vi "BallToGoalSkillVss.vi"(8 "error in (no error)":errorcluster, 9 "Game":refnum<class "Game.lvclass">, 10 "Robot in":refnum<class "Robot.lvclass">, 11 "BallToGoalSkillVSS in":refnum<class "BallToGoalSkillVSS.lvclass">) -> (0 "error out":errorcluster, 2 "Robot out":refnum<class "Robot.lvclass">, 3 "BallToGoalSkillVSS out":refnum<class "BallToGoalSkillVSS.lvclass">)   [LabVIEW 2020, in "BallToGoalSkillVSS.lvclass"]
uses:
  BallToGoalSkillVSS.lvclass
  Robot_class/Robot.lvclass
  C:/Users/pedro/Desktop/SSL_AI/Object_class/Object.lvclass
  Game_class/Game.lvclass
  Game_class/Game.lvclass/Game.ctl
  Object_class/Object.lvclass/Object.ctl
  Robot_class/Robot.lvclass/Robot.ctl
  Game_class/Read BallRef.vi
  Game_class/Read FieldRef.vi
  Object_class/Read x.vi
  Object_class/Read y.vi
  Object_class/Write x.vi
  Object_class/Write y.vi
  Robot_class/Write dest_orientation.vi
  Ball_class/Ball.lvclass
  Field_class/Field.lvclass
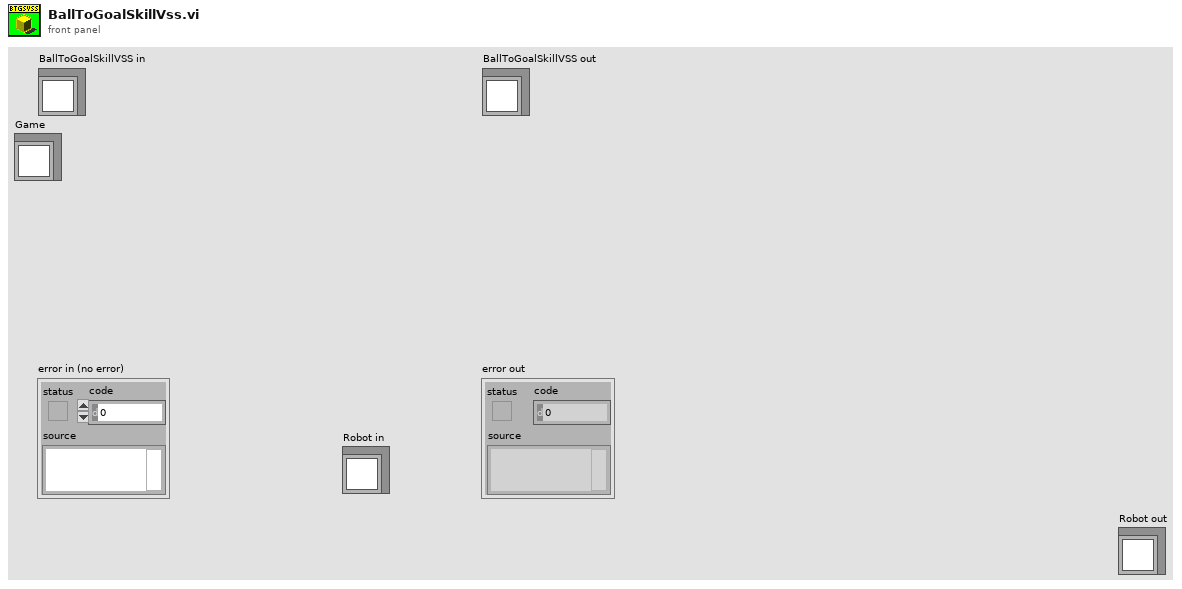
[diagram p1: front panel]
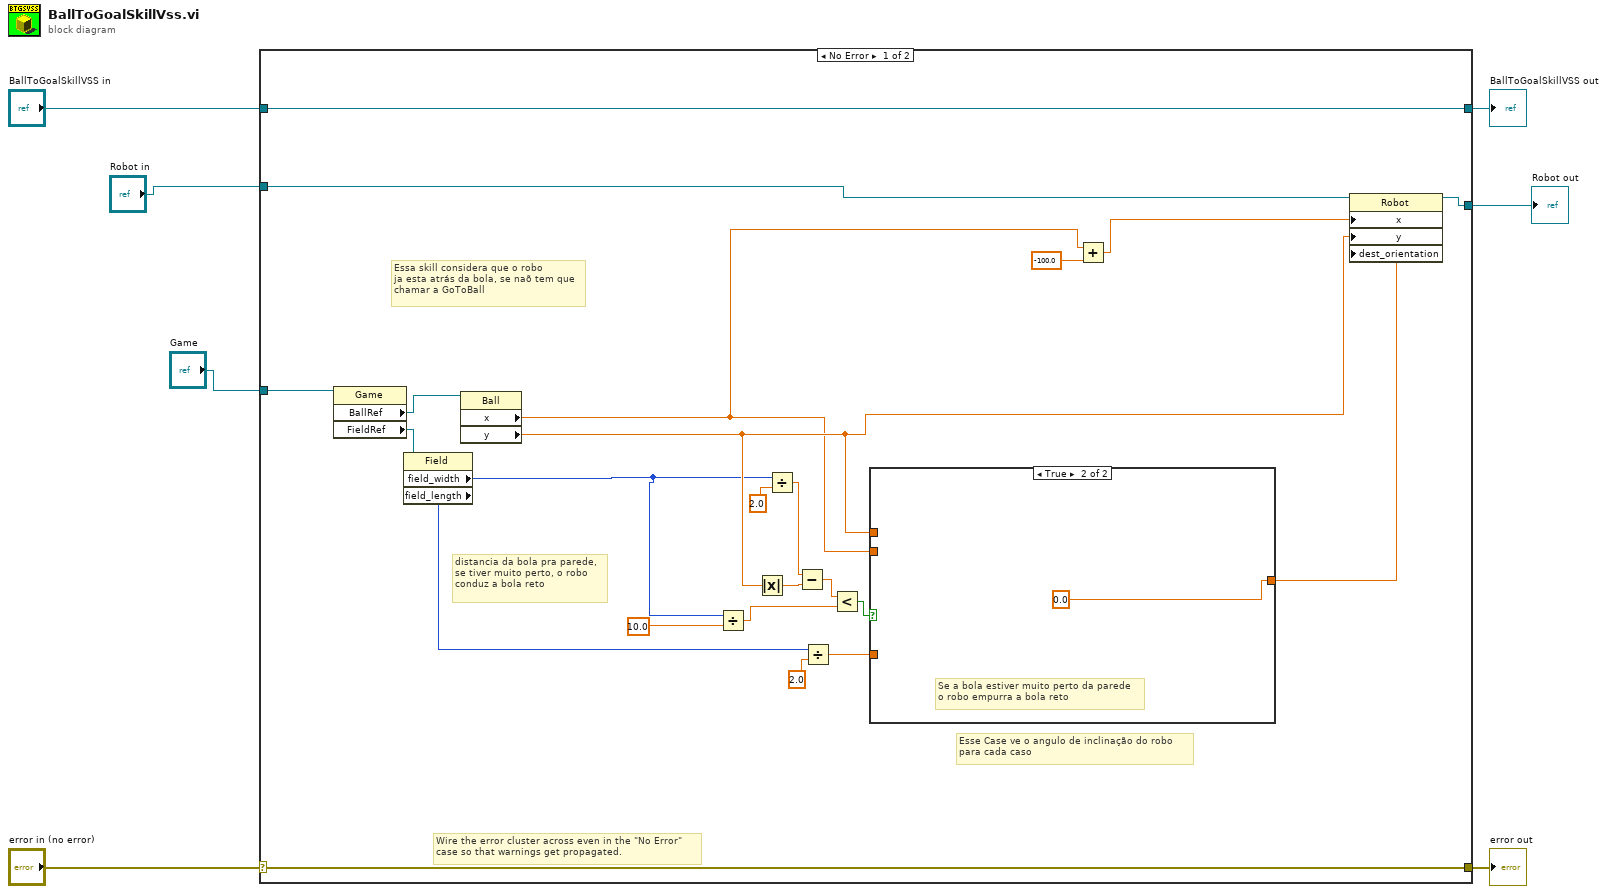
[diagram p0: block diagram]
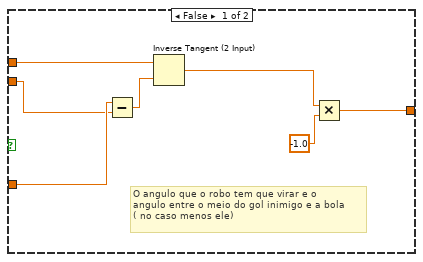
[diagram p2: hidden frame]
diagram:
  n1 = case shown="No Error" "error in (no error)" {
    selector: "error in (no error)" -> [w29 w41]
    tunnel: [w29 w41] -> w6
    tunnel: [w30 w40] -> w4
    tunnel: "BallToGoalSkillVSS in" -> [w30 w40]
    tunnel: "Robot in" -> [w28 w39]
    tunnel: [w24 w39] -> w2
    tunnel: "Game" -> [w27 _]
    frame No Error {
      # "distancia da bola pra parede, se tiver muito perto, o robo conduz a bola reto"
      # "Esse Case ve o angulo de inclinação do robo\npara cada caso"
      # "Essa skill considera que o robo \nja esta atrás da bola, se naõ tem que\nchamar a GoToBall"
      # "Wire the error cluster across even in the \"No Error\"\ncase so that warnings get propagated."
      n2 = property class="Game"(reference=w27) -> ("BallRef"=w26:refnum<class "Ball.lvclass">, "FieldRef"=w25:refnum<class "Field.lvclass">)  [unwired: 1 in, 2 out]
      n3 = property class="Field"(reference=w25) -> ("field_width"=w13:i32, "field_length"=w20:i32)  [unwired: 1 in, 2 out]
      n4 = property class="Ball"(reference=w26) -> ("x"=w9:dbl, "y"=w17:dbl)  [unwired: 1 in, 2 out]
      n5 = Divide(x=w13, y=10.0) -> (x/y=w11:dbl)
      n6 = Absolute Value(x=w17) -> (abs(x)=w16:dbl)
      n7 = Divide(x=w13, y=2.0) -> (x/y=w18:dbl)
      n8 = Subtract(x=w18, y=w16) -> (x-y=w14:dbl)
      n9 = Divide(x=w20, y=2.0) -> (x/y=w22:dbl)
      n10 = Less?(x=w14, y=w11) -> (x < y?=w15:bool)
      n11 = case shown="True" w15 {
        tunnel: w17 -> [w36 _]
        tunnel: w9 -> [w34 _]
        tunnel: w22 -> [w35 _]
        tunnel: [w31 0.0] -> w21
        frame False {
          # "O angulo que o robo tem que virar e o\nangulo entre o meio do gol inimigo e a bola\n( no caso menos ele)"
          n12 = Subtract(x=w35, y=w34) -> (x-y=w33:dbl)
          n13 = Inverse Tangent (2 Input)(1:w33, 2:w36) -> (0:w32:dbl)
          n14 = Multiply(x=w32, y=-1.0) -> (x*y=w31:dbl)
        }
        frame True {
          # "Se a bola estiver muito perto da parede\no robo empurra a bola reto"
        }
      }
      n15 = Add(x=w9, y=-100.0) -> (x+y=w8:dbl)
      n16 = property class="Robot"(reference=w28, "x"=w8, "y"=w17, "dest_orientation"=w21) -> (reference out=w24:refnum<class "Robot.lvclass">)  [unwired: 1 in, 1 out]
    }
    frame Error {
    }
  }
  "error out" <- w6
  "BallToGoalSkillVSS out" <- w4
  "Robot out" <- w2
